vi "sv_Convert Cluster to Array of Variants.vi"(8 "error in (no error)":errorcluster, 11 "cluster in\n(coerced to variant type)":variant) -> (0 "error out":errorcluster, 2 "names":string[](array[string]), 3 "values":variant[](array[variant]))   [LabVIEW 2017]
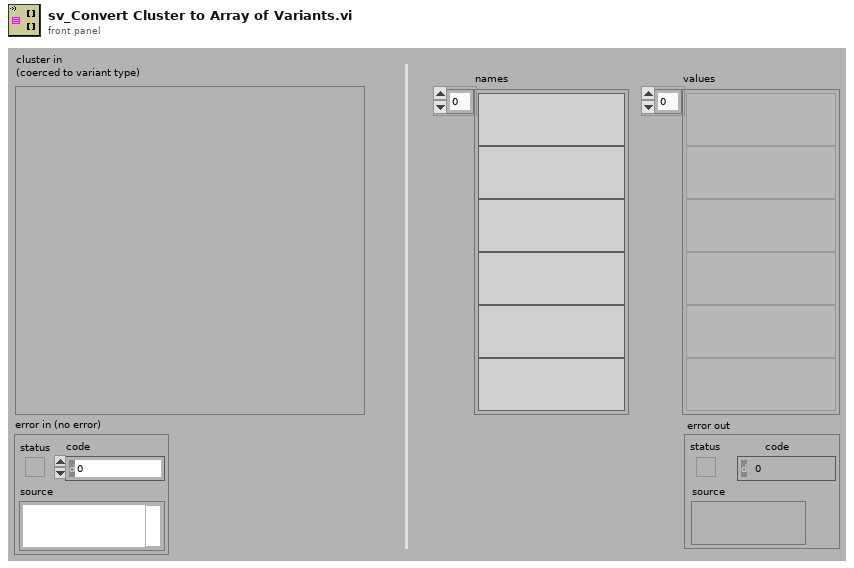
[diagram p1: front panel]
types:
  T1 = cluster{"length":u16, "private":u8, "type":enum8{"<Null>", "I8", "I16", "I32", "I64", "U8", "U16", "U32", "U64", "SGL", "DBL", "EXT", "CSG", "CDB", "CXT", "0x0F", "0x10", "0x11", "0x12", "0x13", "0x14", "Enum U8", "Enum U16", "Enum U32", "Enum U64", "SGL PQ", "DBL PQ", "EXT PQ", "CSG PQ", "CDB PQ", "CXT PQ", "0x1F", "0x20", "Boolean", "0x22", "0x23", "0x24", "0x25", "0x26", "0x27", "0x28", "0x29", "0x2A", "0x2B", "0x2C", "0x2D", "0x2E", "0x2F", "String", "0x31", "Path", "Pict", "0x34", "0x35", "0x36", "DAQ", "0x38", "0x39", "0x3A", "0x3B", "0x3C", "0x3D", "0x3E", "0x3F", "Array", "0x41", "0x42", "0x43", "0x44", "0x45", "0x46", "0x47", "0x48", "0x49", "0x4A", "0x4B", "0x4C", "0x4D", "0x4E", "0x4F", "Cluster", "0x51", "0x52", "Variant", "Waveform", "0x55", "0x56", "0x57", "0x58", "0x59", "0x5A", "0x5B", "0x5C", "0x5D", "0x5E", "0x5F", "0x60", "0x61", "0x62", "0x63", "0x64", "0x65", "0x66", "0x67", "0x68", "0x69", "0x6A", "0x6B", "0x6C", "0x6D", "0x6E", "0x6F", "Refnum"}, "# elements":i32}
  T2 = enum8{"<Null>", "I8", "I16", "I32", "I64", "U8", "U16", "U32", "U64", "SGL", "DBL", "EXT", "CSG", "CDB", "CXT", "0x0F", "0x10", "0x11", "0x12", "0x13", "0x14", "Enum U8", "Enum U16", "Enum U32", "Enum U64", "SGL PQ", "DBL PQ", "EXT PQ", "CSG PQ", "CDB PQ", "CXT PQ", "0x1F", "0x20", "Boolean", "0x22", "0x23", "0x24", "0x25", "0x26", "0x27", "0x28", "0x29", "0x2A", "0x2B", "0x2C", "0x2D", "0x2E", "0x2F", "String", "0x31", "Path", "Pict", "0x34", "0x35", "0x36", "DAQ", "0x38", "0x39", "0x3A", "0x3B", "0x3C", "0x3D", "0x3E", "0x3F", "Array", "0x41", "0x42", "0x43", "0x44", "0x45", "0x46", "0x47", "0x48", "0x49", "0x4A", "0x4B", "0x4C", "0x4D", "0x4E", "0x4F", "Cluster", "0x51", "0x52", "Variant", "Waveform", "0x55", "0x56", "0x57", "0x58", "0x59", "0x5A", "0x5B", "0x5C", "0x5D", "0x5E", "0x5F", "0x60", "0x61", "0x62", "0x63", "0x64", "0x65", "0x66", "0x67", "0x68", "0x69", "0x6A", "0x6B", "0x6C", "0x6D", "0x6E", "0x6F", "Refnum"}
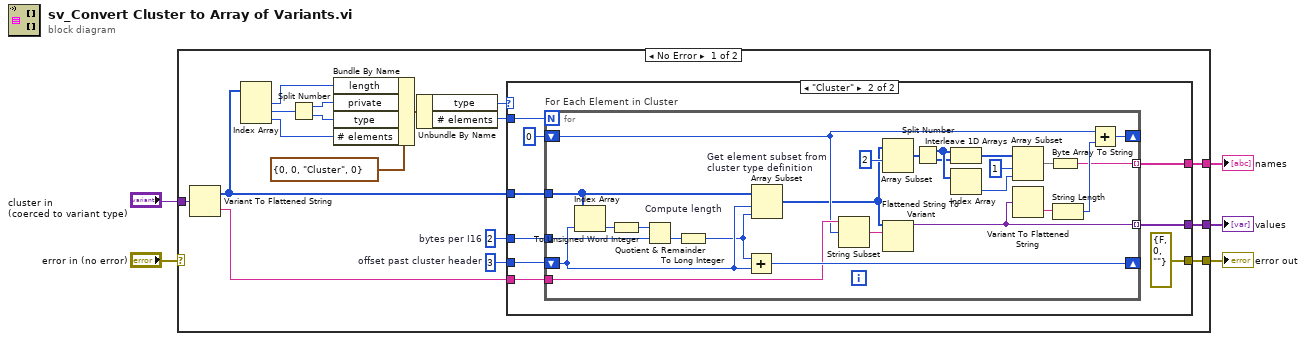
[diagram p0: block diagram]
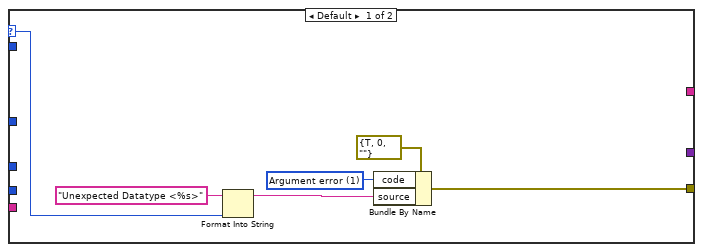
[diagram p2: hidden frame]
diagram:
  n1 = case shown="No Error" "error in (no error)" {
    selector: "error in (no error)" -> [_ w63]
    tunnel: "cluster in\n(coerced to variant type)" -> [w22 _]
    tunnel: [w11 _] -> w4
    tunnel: [w10 w63] -> w3
    tunnel: [w8 _] -> w2
    frame No Error {
      w7 = u16 2  # bytes per I16
      w6 = 3  # offset past cluster header
      n2 = Variant To Flattened String(Variant=w22) -> (data string=w12:string, 1:w16:i16[])
      n3 = Index Array(array=w16) -> (element #1=w18:i16, element #2=w20:i16, element #3=w21:i16)  [unwired: 3 in]
      n4 = Split Number(x=w20) -> (hi(x)=w19:u8, lo(x)=w9:u8)
      n5 = Bundle By Name(cluster=T1 {"length"=0, "private"=0, "type"=enum."Cluster", "# elements"=0} ("Type Descriptor Header"), "length"=w18, "private"=w19, "type"=w9, "# elements"=w21) -> (w13:T1)
      n6 = Unbundle By Name(w13) -> ("type"=w15:T2, "# elements"=w14:i32)
      n7 = case shown="\"Cluster\"" w15 {
        selector: w15 -> [w27 _]
        tunnel: w14 -> [_ w37]
        tunnel: w16 -> [_ w36]
        tunnel: [w25 errorcluster {"status"=FALSE, "code"=0, "source"=""} ("error out")] -> w10
        tunnel: w12 -> [_ w34]
        tunnel: [_ w32] -> w11
        tunnel: [_ w31] -> w8
        tunnel: w7 -> [_ w30]
        tunnel: w6 -> [_ w29]
        frame Default {
          w24 = 1 items=["No error", "Argument error", "Memory is full", "Out of zone", "End of file", "File already open", "Generic file I/O error", "File not found", "File permission error", "Disk is full", "Duplicate path", "Too many files open", "System feature not enabled", "Resource file not found", "Cannot add resource", "Resource not found", "Image not found", "Image memory error", "Pen does not exist", "Config type invalid", "Config token not found", "Config parse error", "Config memory error", "Bad external code format", "Bad external code offset", "External code not present", "Null window", "Destroy window error", "Null menu", "Print aborted", "Bad print record", "Print driver error", "Windows error during printing", "Memory error during printing", "Print dialog error", "Generic print error", "Invalid device refnum", "Device not found", "Device parameter error", "Device unit error", "Cannot open device", "Device call aborted", "Generic error", "Cancelled by user", "Object ID too low", "Object ID too high", "Object not in heap", "Unknown heap", "Unknown object (invalid DefProc)", "Unknown object (DefProc not in table)", "Message out of range", "Invalid (null) method", "Unknown message", "Manager call not supported", "Bad address", "Network operation in progress", "Network operation timed out", "Connection is busy", "Network attribute not supported", "Network error", "Address in use", "System out of memory", "Connection aborted", "Connection refused", "Not connected", "Already connected", "Connection closed", "Initialization error (interapplication manager)", "Bad occurrence", "Wait on unbound occurrence handler", "Occurrence queue overflow", "Datalog type conflict", "Unused", "Unrecognized type (interapplication manager)", "Memory corrupt", "Failed to make temporary DLL", "Old CIN version", "Drag socket not found", "Failed to load drop-object", "Failed to register OLE object", "Failed to release OLE object", "Format specifier type mismatch", "Unknown format specifier", "Too few format specifiers", "Too many format specifiers", "Scan failed", "Newer CIN version", "Error converting to variant", "Runtime menu error", "Password tampered", "Variant attribute not found", "Incompatible variant data type", "Event data is not available", "Event Store is not present", "Occurrence is not found", "Event Queue is not created", "Event info is not available", "Refnum passed is NULL", "Error retrieving Class GUID", "Error retrieving CoClass GUID", "Error retrieving TypeLib GUID.", "Bad built application magic bytes.", "Specific driver is different from the specific driver associated with the Logical Name.", "There is no session opened to the class driver.", "Max Error", "MAX - Error with config objects", "MAX - Error loading configuration", "MAX - Group not supported"]
          n8 = Format Into String(format string="Unexpected Datatype <%s>" ("Format String"), w27) -> (resulting string=w23:string)  [unwired: 2 in, 1 out]
          n9 = Bundle By Name(cluster=errorcluster {"status"=TRUE, "code"=0, "source"=""} ("error out"), "code"=w24, "source"=w23) -> (w25:errorcluster)
        }
        frame "Cluster" {
          n10 = for "For Each Element in Cluster" {
            N: w37 -> [_]
            shift-right: [w61] -> _
            shift-left: w29 -> [w60]
            tunnel: w36 -> [w62]
            tunnel: w34 -> [w52]
            shift-right: [w51] -> _
            shift-left: 0 -> [w50]
            tunnel: [w49] -> w32 mode=indexing
            tunnel: w30 -> [w48]
            tunnel: [w38] -> w31 mode=indexing
            n11 = Index Array(array=w62, index=w60) -> (element=w58:i16)
            n12 = To Unsigned Word Integer(number=w58) -> (unsigned 16bit integer=w57:u16)
            n13 = Quotient & Remainder "Compute length"(x=w57, y=w48) -> (floor(x/y)=w59:u16)  [unwired: 1 out]
            n14 = To Long Integer(number=w59) -> (32bit integer=w56:i32)
            n15 = Add(x=w56, y=w60) -> (x+y=w61:i32)
            n16 = Array Subset "Get element subset from cluster type definition"(array=w62, index=w60, length=w56) -> (w39:i16[])
            n17 = String Subset(string=w52, offset (0)=w50) -> (substring=w54:string)  [unwired: 1 in]
            n18 = Array Subset(array=w39, index=2) -> (w44:i16[])  [unwired: 1 in]
            n19 = Flattened String To Variant(6:w54, 7:w39) -> (3:w49:variant)  [unwired: 1 in, 1 out]
            n20 = Split Number(x=w44) -> (hi(x)=w42:u8[], lo(x)=w41:u8[])
            n21 = Interleave 1D Arrays(w42, w41) -> (w40:u8[])
            n22 = Index Array(array=w42) -> (element=w43:u8)  [unwired: 1 in]
            n23 = Array Subset(array=w40, index=1, length=w43) -> (w45:u8[])
            n24 = Variant To Flattened String(Variant=w49) -> (data string=w53:string)  [unwired: 1 out]
            n25 = Byte Array To String(unsigned byte array=w45) -> (string=w38:string)
            n26 = String Length(string=w53) -> (length=w55:i32)
            n27 = Add(x=w50, y=w55) -> (x+y=w51:i32)
          }
        }
      }
    }
    frame Error {
    }
  }
  "values" <- w4
  "error out" <- w3
  "names" <- w2
